vi "Set Pod Setpoints NEO.vi"(8 "Steer Angles (degrees)":T2, 9 "Drive Velocities (ft/s)":T2, 10 "Pod Setpoints (ft/s and deg)":T12, 11 "Motors":T4={"Drive Motors"={"Motor Type"=enum."Falcon 500", "Motors"={"Left Front"={"DeviceStatus"={"status"=FALSE, "code"=0, "source"=""}, "Type"=enum."PWM", "PWM"={"PWM Channel"=enum."PWM 0", "DeadBand"={"Name"="", "maxPositivePwm"=0, "minPositivePwm"=0, "centerPwm"=0, "maxNegativePwm"=0, "minNegativePwm"=0, "angularRange"=0}}, "CAN"={"Device Number"=0, "SetOutput VI Ref"=variant, "GetOutput VI Ref"=variant, "Enable VI Ref"=variant, "Disable VI Ref"=variant, "Data"=variant}, "Invert"=FALSE, "DIO PWM"={"PWM \"Enable\" Channel"=enum."PWM 0", "DIOChannel"=enum."DIO 0", "PWM Rate"=0.0}}, "Left Back"={"DeviceStatus"={"status"=FALSE, "code"=0, "source"=""}, "Type"=enum."PWM", "PWM"={"PWM Channel"=enum."PWM 0", "DeadBand"={"Name"="", "maxPositivePwm"=0, "minPositivePwm"=0, "centerPwm"=0, "maxNegativePwm"=0, "minNegativePwm"=0, "angularRange"=0}}, "CAN"={"Device Number"=0, "SetOutput VI Ref"=variant, "GetOutput VI Ref"=variant, "Enable VI Ref"=variant, "Disable VI Ref"=variant, "Data"=variant}, "Invert"=FALSE, "DIO PWM"={"PWM \"Enable\" Channel"=enum."PWM 0", "DIOChannel"=enum."DIO 0", "PWM Rate"=0.0}}, "Right Front"={"DeviceStatus"={"status"=FALSE, "code"=0, "source"=""}, "Type"=enum."PWM", "PWM"={"PWM Channel"=enum."PWM 0", "DeadBand"={"Name"="", "maxPositivePwm"=0, "minPositivePwm"=0, "centerPwm"=0, "maxNegativePwm"=0, "minNegativePwm"=0, "angularRange"=0}}, "CAN"={"Device Number"=0, "SetOutput VI Ref"=variant, "GetOutput VI Ref"=variant, "Enable VI Ref"=variant, "Disable VI Ref"=variant, "Data"=variant}, "Invert"=FALSE, "DIO PWM"={"PWM \"Enable\" Channel"=enum."PWM 0", "DIOChannel"=enum."DIO 0", "PWM Rate"=0.0}}, "Right Back"={"DeviceStatus"={"status"=FALSE, "code"=0, "source"=""}, "Type"=enum."PWM", "PWM"={"PWM Channel"=enum."Invalid", "DeadBand"={"Name"="", "maxPositivePwm"=0, "minPositivePwm"=0, "centerPwm"=0, "maxNegativePwm"=0, "minNegativePwm"=0, "angularRange"=0}}, "CAN"={"Device Number"=0, "SetOutput VI Ref"=variant, "GetOutput VI Ref"=variant, "Enable VI Ref"=variant, "Disable VI Ref"=variant, "Data"=variant}, "Invert"=FALSE, "DIO PWM"={"PWM \"Enable\" Channel"=enum."Invalid", "DIOChannel"=enum."Invalid", "PWM Rate"=0.0}}}}, "Steering Motors"={"Motor Type"=enum."Falcon 500", "Motors"={"Left Front"={"DeviceStatus"={"status"=FALSE, "code"=0, "source"=""}, "Type"=enum."PWM", "PWM"={"PWM Channel"=enum."PWM 0", "DeadBand"={"Name"="", "maxPositivePwm"=0, "minPositivePwm"=0, "centerPwm"=0, "maxNegativePwm"=0, "minNegativePwm"=0, "angularRange"=0}}, "CAN"={"Device Number"=0, "SetOutput VI Ref"=variant, "GetOutput VI Ref"=variant, "Enable VI Ref"=variant, "Disable VI Ref"=variant, "Data"=variant}, "Invert"=FALSE, "DIO PWM"={"PWM \"Enable\" Channel"=enum."PWM 0", "DIOChannel"=enum."DIO 0", "PWM Rate"=0.0}}, "Left Back"={"DeviceStatus"={"status"=FALSE, "code"=0, "source"=""}, "Type"=enum."PWM", "PWM"={"PWM Channel"=enum."PWM 0", "DeadBand"={"Name"="", "maxPositivePwm"=0, "minPositivePwm"=0, "centerPwm"=0, "maxNegativePwm"=0, "minNegativePwm"=0, "angularRange"=0}}, "CAN"={"Device Number"=0, "SetOutput VI Ref"=variant, "GetOutput VI Ref"=variant, "Enable VI Ref"=variant, "Disable VI Ref"=variant, "Data"=variant}, "Invert"=FALSE, "DIO PWM"={"PWM \"Enable\" Channel"=enum."PWM 0", "DIOChannel"=enum."DIO 0", "PWM Rate"=0.0}}, "Right Front"={"DeviceStatus"={"status"=FALSE, "code"=0, "source"=""}, "Type"=enum."PWM", "PWM"={"PWM Channel"=enum."PWM 0", "DeadBand"={"Name"="", "maxPositivePwm"=0, "minPositivePwm"=0, "centerPwm"=0, "maxNegativePwm"=0, "minNegativePwm"=0, "angularRange"=0}}, "CAN"={"Device Number"=0, "SetOutput VI Ref"=variant, "GetOutput VI Ref"=variant, "Enable VI Ref"=variant, "Disable VI Ref"=variant, "Data"=variant}, "Invert"=FALSE, "DIO PWM"={"PWM \"Enable\" Channel"=enum."PWM 0", "DIOChannel"=enum."DIO 0", "PWM Rate"=0.0}}, "Right Back"={"DeviceStatus"={"status"=FALSE, "code"=0, "source"=""}, "Type"=enum."PWM", "PWM"={"PWM Channel"=enum."Invalid", "DeadBand"={"Name"="", "maxPositivePwm"=0, "minPositivePwm"=0, "centerPwm"=0, "maxNegativePwm"=0, "minNegativePwm"=0, "angularRange"=0}}, "CAN"={"Device Number"=0, "SetOutput VI Ref"=variant, "GetOutput VI Ref"=variant, "Enable VI Ref"=variant, "Disable VI Ref"=variant, "Data"=variant}, "Invert"=FALSE, "DIO PWM"={"PWM \"Enable\" Channel"=enum."Invalid", "DIOChannel"=enum."Invalid", "PWM Rate"=0.0}}}}}) -> ()   [LabVIEW 2020]
uses:
  ctl/Pod Setpoints.ctl
  ctl/Swerve Motors.ctl
  ctl/4 Motor Set.ctl
  ctl/Motor Type.ctl
  <vilib>/Rock Robotics/WPI/MotorControl/WPI_MotorControlDeviceRef.ctl
  <vilib>/Rock Robotics/WPI/MotorControl/WPI_MotorControlType.ctl
  <vilib>/Rock Robotics/SystemInterfaces/DIO/FPGA_DIOPWMChannel.ctl
  <vilib>/Rock Robotics/WPI/PWM/WPI_PWMDeadband.ctl
  <vilib>/Rock Robotics/SystemInterfaces/DIO/FPGA_DIOChannel.ctl
  <vilib>/Rock Robotics/WPI/ThirdParty/Phoenix-LabVIEW/Motor Controller/Controls/CTRE_Phoenix_MotorControl_ControlMode.ctl
panel:
  in  "PID Constants":T1={"P Gain"=0.0, "I Gain"=0.0, "D Gain"=0.0, "F Gain"=0.0, "I Zone"=0.0, "Min Output"=-1.0, "Max Output"=1.0}
  out "Updated":bool
  in  "Push PID":bool
  out "PID Graph":cluster{"Left Front":i32, "Theta":dbl}(graph)
  in  "Motor Position":T3(ring)
  in  "Motor Type":enum16{"Drive", "Steer"}(ring)
  in  "Debug Mode?":bool
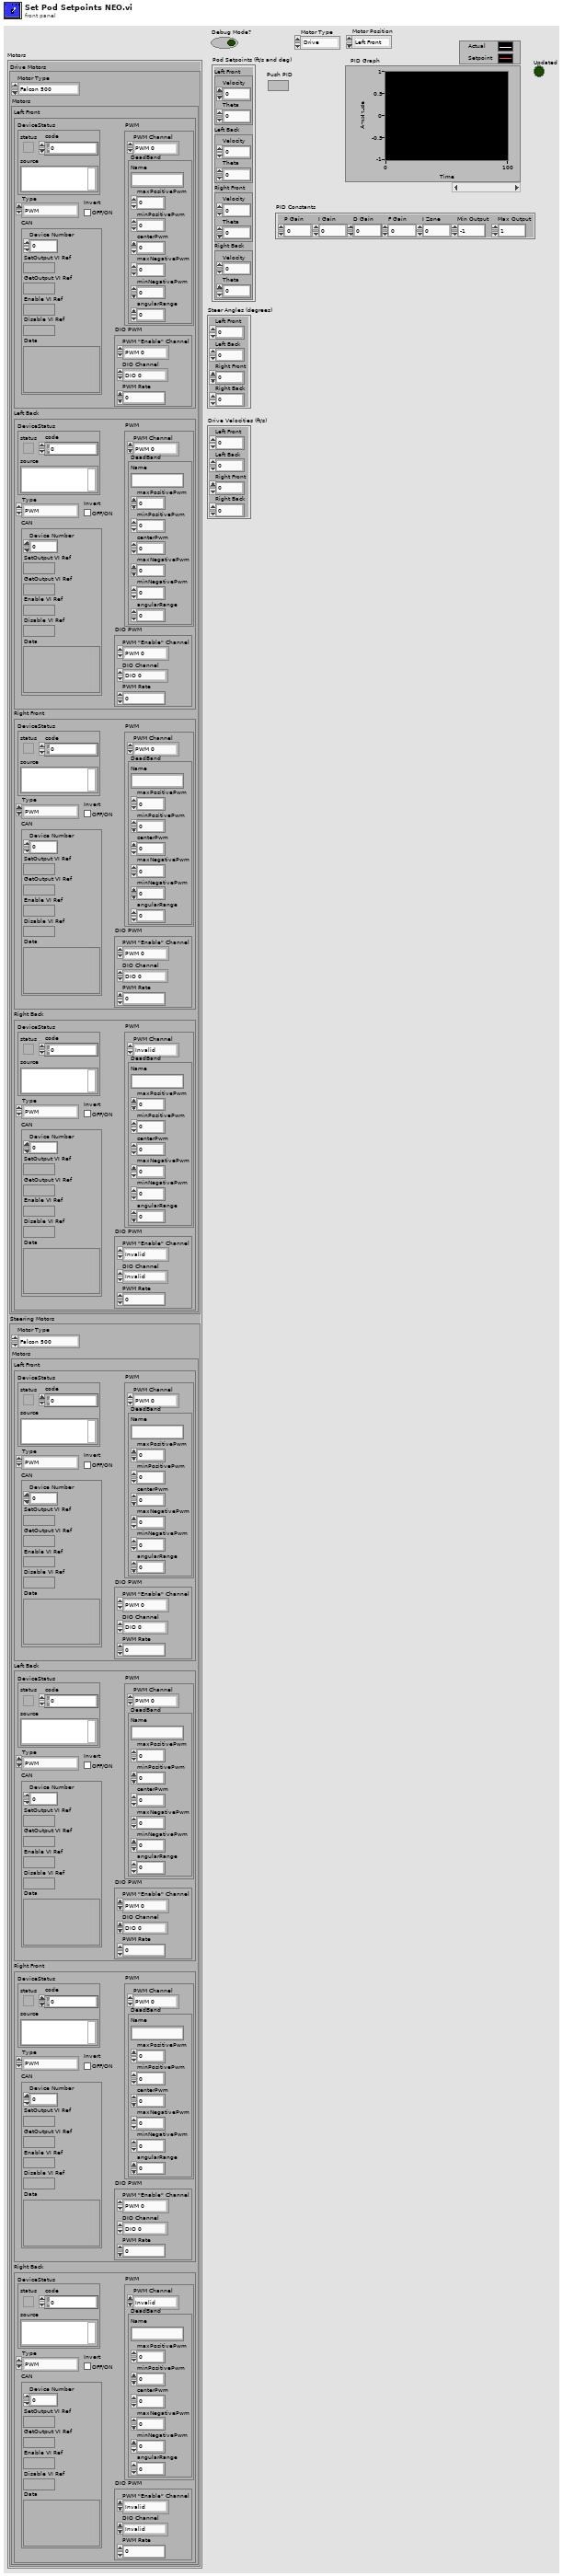
[diagram p1: front panel]
types:
  T1 = cluster{"P Gain":dbl, "I Gain":dbl, "D Gain":dbl, "F Gain":dbl, "I Zone":dbl, "Min Output":dbl, "Max Output":dbl}
  T2 = cluster{"Left Front":i32, "Left Back":i32, "Right Front":i32, "Right Back":i32}
  T3 = enum16{"Left Front", "Left Back", "Right Front", "Right Back"}
  T4 = typedef "Swerve Motors.ctl" = cluster{"Drive Motors":T5, "Steering Motors":T5}
  T5 = typedef "4 Motor Set.ctl" = cluster{"Motor Type":T6, "Motors":cluster{"Left Front":T7, "Left Back":T7, "Right Front":T7, "Right Back":T7}}
  T6 = typedef "Motor Type.ctl" = enum16{"Falcon 500", "NEO", "NEO 550"}
  T7 = typedef "WPI_MotorControlDeviceRef.ctl" = cluster{"DeviceStatus":errorcluster, "Type":T8, "PWM":cluster{"PWM Channel":T9, "DeadBand":T10}, "CAN":cluster{"Device Number":u8, "SetOutput VI Ref":variant, "GetOutput VI Ref":variant, "Enable VI Ref":variant, "Disable VI Ref":variant, "Data":variant}, "Invert":bool, "DIO PWM":cluster{"PWM \"Enable\" Channel":T9, "DIOChannel":T11, "PWM Rate":dbl}}
  T8 = typedef "WPI_MotorControlType.ctl" = enum16{"PWM", "CAN", "DIO PWM"}
  T9 = typedef "FPGA_DIOPWMChannel.ctl" = enum8{"PWM 0", "PWM 1", "PWM 2", "PWM 3", "PWM 4", "PWM 5", "PWM 6", "PWM 7", "PWM 8", "PWM 9", "PWM MXP 0", "PWM MXP 1", "PWM MXP 2", "PWM MXP 3", "PWM MXP 4", "PWM MXP 5", "PWM MXP 6", "PWM MXP 7", "PWM MXP 8", "PWM MXP 9", "Invalid"}
  T10 = typedef "WPI_PWMDeadband.ctl" = cluster{"Name":string, "maxPositivePwm":i32, "minPositivePwm":i32, "centerPwm":i32, "maxNegativePwm":i32, "minNegativePwm":i32, "angularRange":u16}
  T11 = typedef "FPGA_DIOChannel.ctl" = enum8{"DIO 0", "DIO 1", "DIO 2", "DIO 3", "DIO 4", "DIO 5", "DIO 6", "DIO 7", "DIO 8", "DIO 9", "DIO MXP 0", "DIO MXP 1", "DIO MXP 2", "DIO MXP 3", "DIO MXP 4", "DIO MXP 5", "DIO MXP 6", "DIO MXP 7", "DIO MXP 8", "DIO MXP 9", "DIO MXP 10", "DIO MXP 11", "DIO MXP 12", "DIO MXP 13", "DIO MXP 14", "DIO MXP 15", "SPI Port CS1", "SPI Port CS2", "SPI Port CS3", "SPI Port MISO", "SPI Port MOSI", "Invalid"}
  T12 = typedef "Pod Setpoints.ctl" = cluster{"Left Front":cluster{"Velocity":dbl, "Theta":dbl}, "Left Back":cluster{"Velocity":dbl, "Theta":dbl}, "Right Front":cluster{"Velocity":dbl, "Theta":dbl}, "Right Back":cluster{"Velocity":dbl, "Theta":dbl}}
  T13 = typedef "CTRE_Phoenix_MotorControl_ControlMode.ctl" = u16
  T14 = cluster{"Left Front":T7, "Left Back":T7, "Right Front":T7, "Right Back":T7}
  T15 = cluster{"[0]":dbl, "[1]":dbl, "[2]":dbl, "[3]":dbl}
  T16 = cluster{"Left Front":dbl, "Left Back":dbl, "Right Front":dbl, "Right Back":dbl}
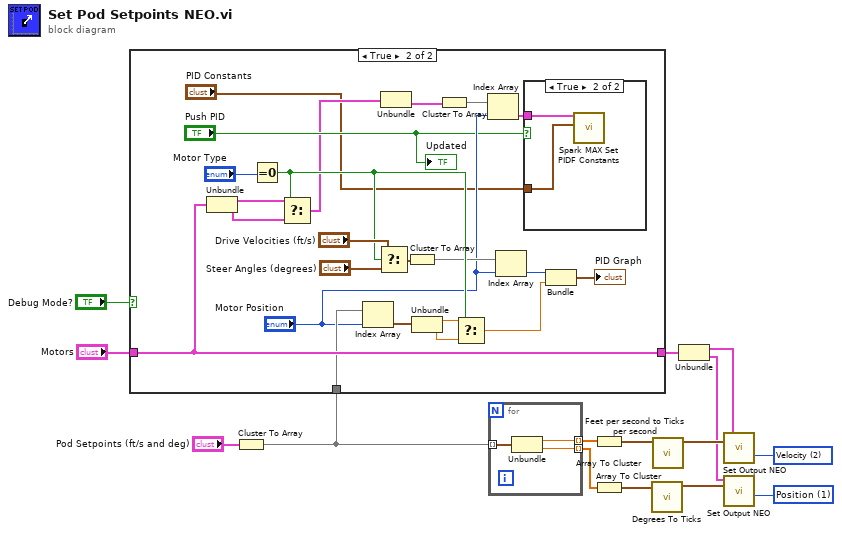
[diagram p0: block diagram]
diagram:
  w1 = T13 1 items=["PercentOutput"=0, "Position"=1, "Velocity"=2, "Current"=3, "Follower"=5, "MotionProfile"=6, "MotionMagic"=7, "MotionProfileArc"=10, "Disabled"=15] ("Control Mode")
  w4 = T13 2 items=["PercentOutput"=0, "Position"=1, "Velocity"=2, "Current"=3, "Follower"=5, "MotionProfile"=6, "MotionMagic"=7, "MotionProfileArc"=10, "Disabled"=15] ("Control Mode")
  n1 = Cluster To Array(cluster="Pod Setpoints (ft/s and deg)") -> (array=w7:cluster{"Velocity":dbl, "Theta":dbl}[])
  n2 = case shown="True" "Debug Mode?" {
    tunnel: "Motors" -> [w16 w39]
    tunnel: [w16 w39] -> w9
    tunnel: w7 -> [_ w35]
    frame False {
    }
    frame True {
      n3 = Unbundle(w39) -> ("Drive Motors"=w37:T5, "Steering Motors"=w36:T5)
      n4 = Equal To 0?(x="Motor Type") -> (x = 0?=w27:bool)
      n5 = Select(t=w37, s=w27, f=w36) -> (s? t:f=w19:T5)
      n6 = Index Array(array=w35, index="Motor Position") -> (element=w34:cluster{"Velocity":dbl, "Theta":dbl})
      n7 = Select(t="Drive Velocities (ft/s)", s=w27, f="Steer Angles (degrees)") -> (s? t:f=w26:T2)
      n8 = Unbundle(w19) -> ("Motors"=w18:T14)  [unwired: 1 out]
      n9 = Cluster To Array(cluster=w26) -> (array=w25:i32[])
      n10 = Unbundle(w34) -> ("Velocity"=w33:dbl, "Theta"=w32:dbl)
      n11 = Cluster To Array(cluster=w18) -> (array=w23:T7[])
      n12 = Select(t=w33, s=w27, f=w32) -> (s? t:f=w31:dbl)
      n13 = Index Array(array=w23, index="Motor Position") -> (element=w21:T7)
      n14 = Index Array(array=w25, index="Motor Position") -> (element=w24:i32)
      n15 = case shown="True" "Push PID" {
        tunnel: w21 -> [_ w40]
        tunnel: "PID Constants" -> [_ w41]
        frame False {
        }
        frame True {
          n16 = call <vilib>:"Spark MAX Set PIDF Constants.vi"("PID Constants"=w41, "MotorControlDeviceRef"=w40) -> ()  [unwired: 8 in, 2 out]
        }
      }
      n17 = Bundle("Left Front"=w24, "Theta"=w31) -> (→"PID Graph":cluster{"Left Front":i32, "Theta":dbl})  [unwired: 1 in]
      "Updated" <- "Push PID"
    }
  }
  n18 = for {
    tunnel: w7 -> [w44] mode=indexing
    tunnel: [w43] -> w15 mode=indexing
    tunnel: [w42] -> w14 mode=indexing
    n19 = Unbundle(w44) -> ("Velocity"=w43:dbl, "Theta"=w42:dbl)
  }
  n20 = Array To Cluster(array=w15) -> (cluster=w12:T15)
  n21 = Array To Cluster(array=w14) -> (cluster=w13:T15)
  n22 = call "Degrees To Ticks.vi"("Steering Angles (degrees)"=w13) -> ("Steering Angles (ticks)"=w2:T16)  [unwired: 10 in]
  n23 = call "Feet per second to Ticks per second.vi"("Drive Velocities (ft/s)"=w12) -> ("Drive Velocities (ticks/ds)"=w5:T16)  [unwired: 10 in]
  n24 = Unbundle(w9) -> ("Drive Motors"=w6:T5, "Steering Motors"=w3:T5)
  n25 = call "Set Output NEO.vi"("Control Mode"=w4, "Setpoints"=w5, "Motors"=w6) -> ()  [unwired: 9 in]
  n26 = call "Set Output NEO.vi"("Control Mode"=w1, "Setpoints"=w2, "Motors"=w3) -> ()  [unwired: 9 in]
